vi "AH_PreCMD.vi"(8 "error in (no error)":errorcluster, 9 "CMD":string, 10 "Data Cluster In":T1 {"GUI Data Cluster"."SBR" format="%08b"}, 11 "Config Cluster In":T3={"General"={"Config.ini"=path "", "Default Logging Path"=path ""}, "Hardware"={"Global T VAR"="", "Global B VAR"="", "VISAS"={"GEN COM"="", "SCOPE COM"="", "VNA COM"=""}, "Connected?"={"SCOPE"=FALSE, "GEN"=FALSE, "VNA"=FALSE}}, "Operation"={"Operation Mode"=enum."Logging", "Status"="", "NewLog?"=FALSE, "OvenWarn"=FALSE, "Scope Settings"={"TimeBase"=0.0, "VerticalScale"=4.0}}}) -> (0 "error IO":errorcluster, 2 "Data Cluster Out":T1 {"GUI Data Cluster"."SBR" format="%08b"}, 3 "Configuration Cluster Out":T3={"General"={"Config.ini"=path "", "Default Logging Path"=path ""}, "Hardware"={"Global T VAR"="", "Global B VAR"="", "VISAS"={"GEN COM"="", "SCOPE COM"="", "VNA COM"=""}, "Connected?"={"SCOPE"=FALSE, "GEN"=FALSE, "VNA"=FALSE}}, "Operation"={"Operation Mode"=enum."Idle-Off", "Status"="", "NewLog?"=FALSE, "OvenWarn"=FALSE, "Scope Settings"={"TimeBase"=0.0, "VerticalScale"=4.0}}})   [LabVIEW 2021]
uses:
  Mode_Enum.ctl
  Config_Cluster.ctl
  Measurement_Cluster.ctl
  Data_Cluster.ctl
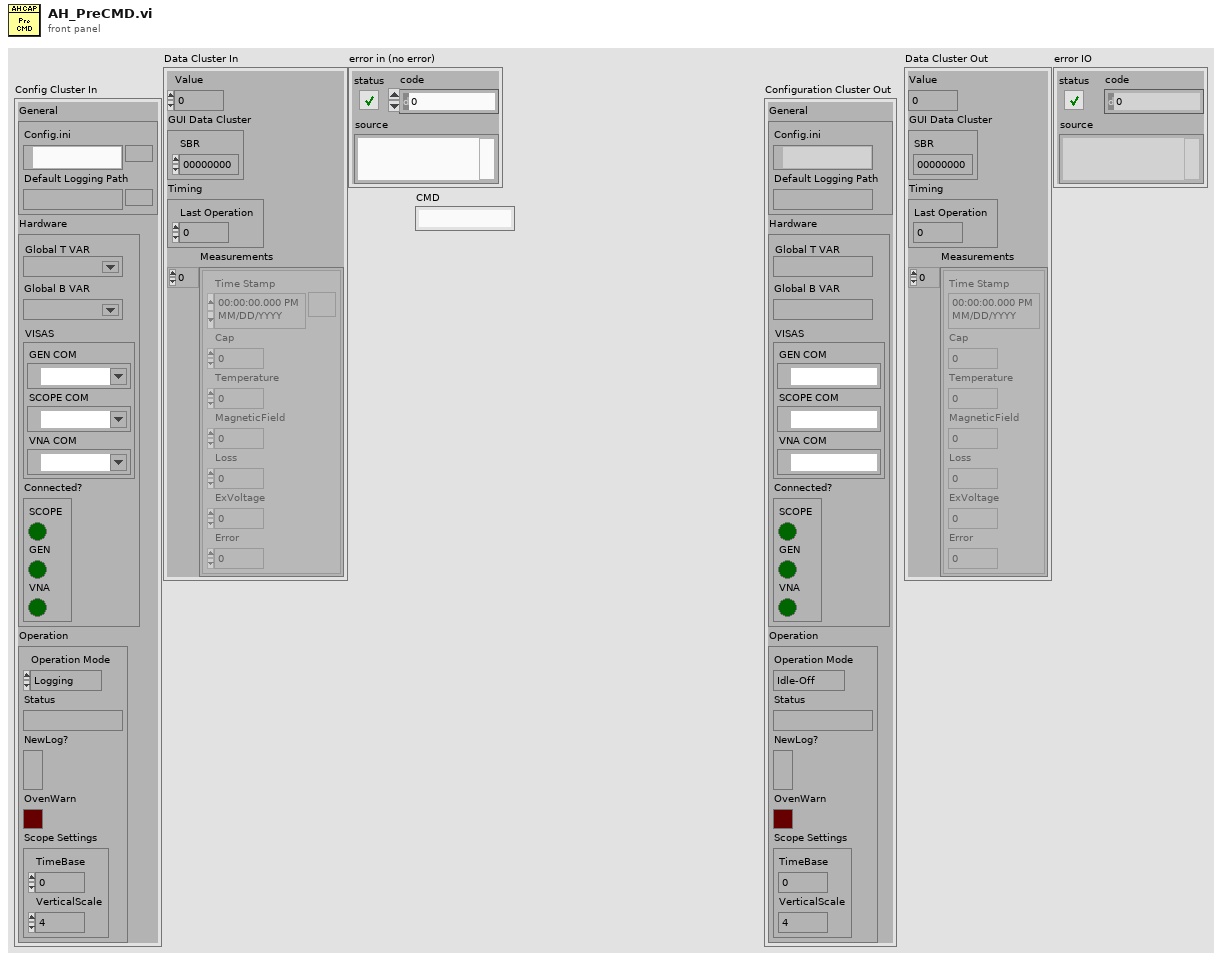
[diagram p1: front panel]
types:
  T1 = typedef "Data_Cluster.ctl" = cluster{"Value":dbl, "GUI Data Cluster":cluster{"SBR":u16}, "Timing":cluster{"Last Operation":dbl}, "Measurements":T2[]}
  T2 = typedef "Measurement_Cluster.ctl" = cluster{"Time Stamp":timestamp, "Cap":dbl, "Temperature":dbl, "MagneticField":dbl, "Loss":dbl, "ExVoltage":dbl, "Error":dbl}
  T3 = typedef "Config_Cluster.ctl" = cluster{"General":cluster{"Config.ini":path, "Default Logging Path":path}, "Hardware":cluster{"Global T VAR":refnum<k21>, "Global B VAR":refnum<k21>, "VISAS":cluster{"GEN COM":refnum<visa-resource-name>, "SCOPE COM":refnum<visa-resource-name>, "VNA COM":refnum<visa-resource-name>}, "Connected?":cluster{"SCOPE":bool, "GEN":bool, "VNA":bool}}, "Operation":cluster{"Operation Mode":T4, "Status":string, "NewLog?":bool, "OvenWarn":bool, "Scope Settings":cluster{"TimeBase":dbl, "VerticalScale":dbl}}}
  T4 = typedef "Mode_Enum.ctl" = enum16{"OvenNRDY", "Logging", "Idle-Off", "Idle"}
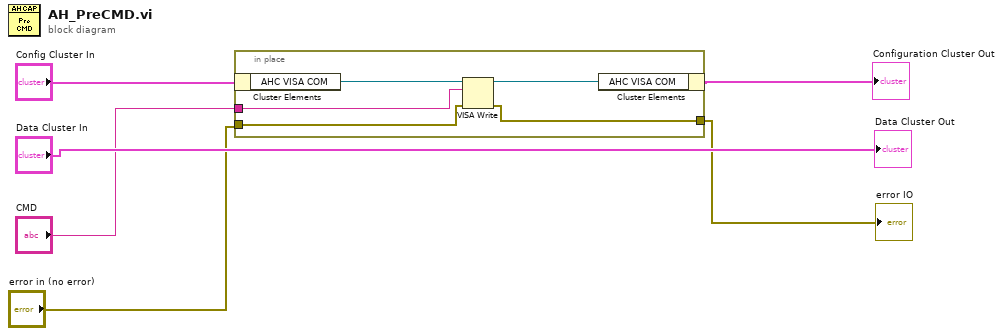
[diagram p0: block diagram]
diagram:
  n1 = in-place {
    in-place-border: "error in (no error)" -> [w9]
    in-place-border: [w8] -> w2
    in-place-border: "CMD" -> [w7]
    n2 = in-place-cluster #1("Config Cluster In") -> ("AHC VISA COM"=w11:refnum<visa-resource-name>)
    n3 = VISA Write(VISA resource name=w11, write buffer=w7, error in (no error)=w9) -> (VISA resource name out=w10:refnum<visa-resource-name>, error out=w8:errorcluster)  [unwired: 1 out]
    n4 = in-place-cluster #1("AHC VISA COM"=w10) -> (→"Configuration Cluster Out":T3)
  }
  "error IO" <- w2
  "Data Cluster Out" <- "Data Cluster In"
